vi "MakePhiAxis (SubVI).vi"(2 "radialBinAxis":dbl[](array[numeric]), 3 "angular pixel \ncoverage factor":dbl) -> (15 "lengths":i32[](array[numeric]), 16 "Rsin(phi)[Q]":dbl[][][](array[numeric]), 17 "Rcos(phi)[Q]":dbl[][][](array[numeric]))   [LabVIEW 2011, in "OfflineTracker.lvlib"]
uses:
  OfflineTracker.lvlib
panel:
  out "Waveform Graph":dbl[][](graph)
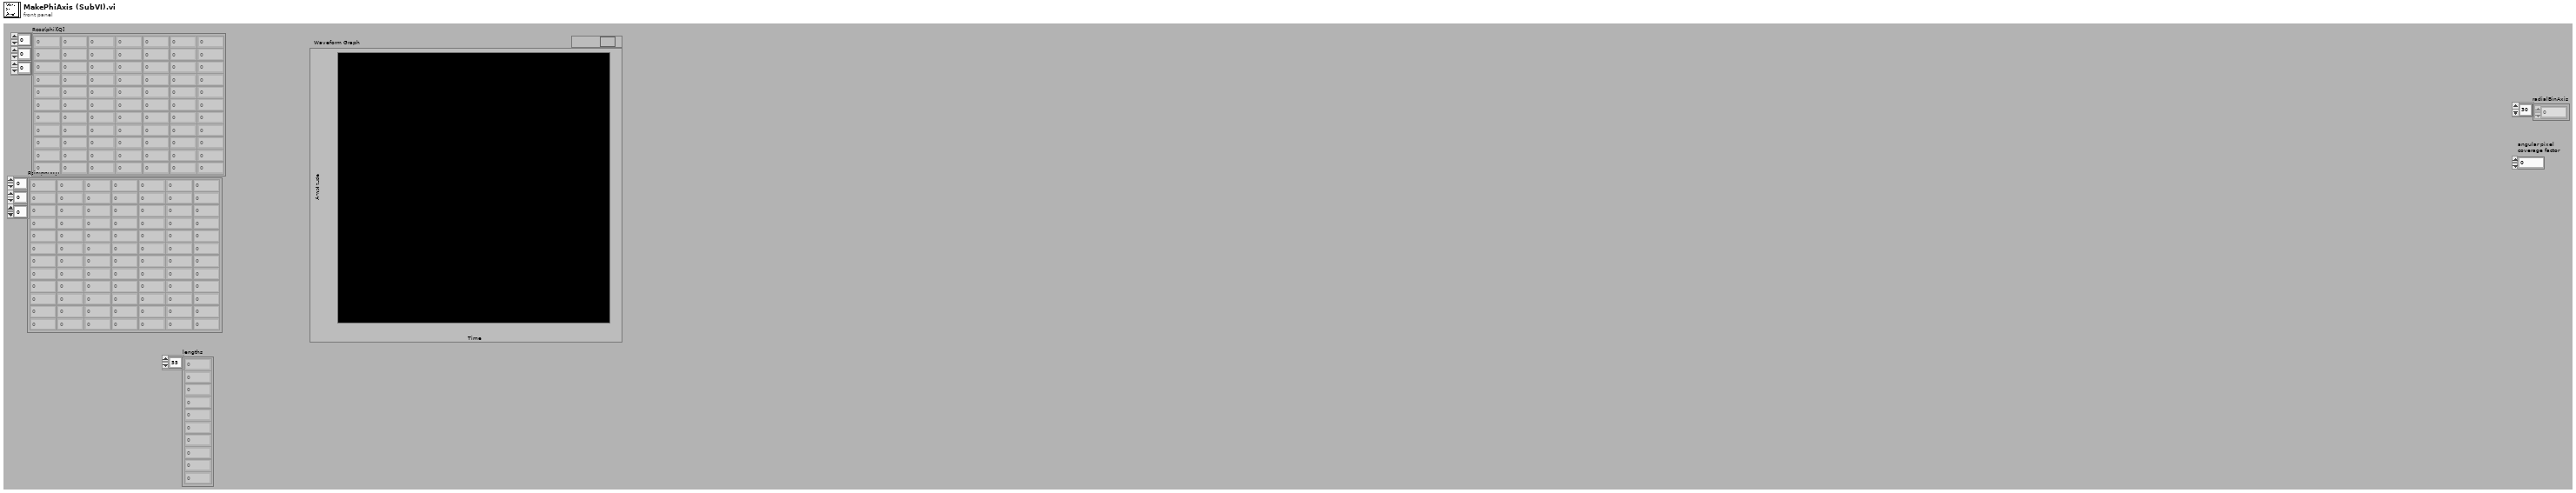
[diagram p1: front panel]
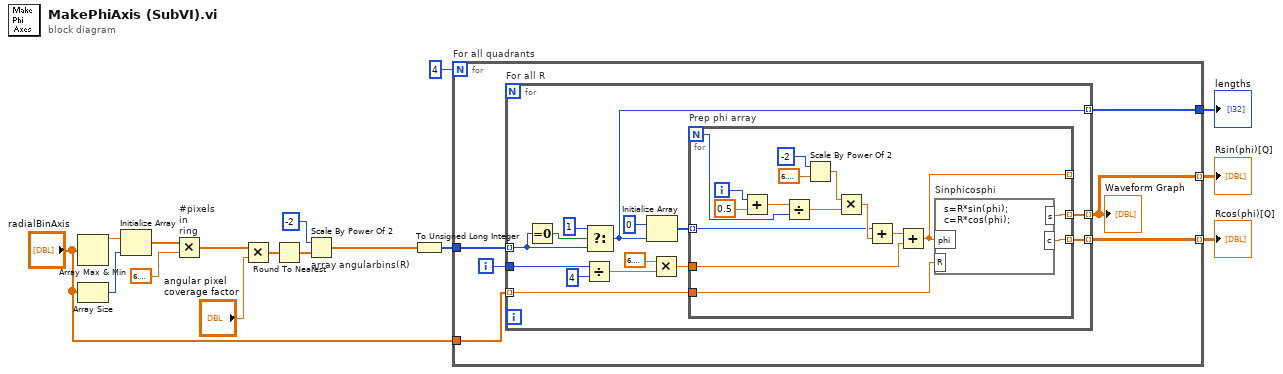
[diagram p0: block diagram]
diagram:
  n1 = Array Max & Min(array="radialBinAxis") -> (max value=w2:dbl)  [unwired: 3 out]
  n2 = Array Size(array="radialBinAxis") -> (size(s)=w3:i32)
  n3 = Initialize Array(w2, w3) -> (w1:dbl[])
  n4 = Multiply "#pixels\nin\nring"(x=w1, y=6.283185307179586) -> (x*y=w9:dbl[])
  n5 = Multiply(x=w9, y="angular pixel \ncoverage factor") -> (x*y=w8:dbl[])
  n6 = Round To Nearest(number=w8) -> (nearest integer value=w7:dbl[])
  n7 = Scale By Power Of 2 "array angularbins(R)"(n=-2, x=w7) -> (x*2^n=w14:dbl[])
  n8 = To Unsigned Long Integer(number=w14) -> (unsigned 32bit integer=w6:u32[])
  n9 = for "For all quadrants" {
    N: 4 -> [_]
    tunnel: w6 -> [w22]
    tunnel: [w19] -> w10 mode=indexing
    tunnel: [w21] -> w11 mode=indexing
    tunnel: "radialBinAxis" -> [w20]
    tunnel: [w17] -> w5
    i -> [w18]
    n10 = for "For all R" {
      tunnel: w22 -> [w24] mode=indexing
      tunnel: [w29] -> w21 mode=indexing
      tunnel: [w30] -> w19 mode=indexing
      tunnel: w18 -> [w28]
      tunnel: w20 -> [w27] mode=indexing
      tunnel: [w23] -> w17 mode=indexing
      n11 = Equal To 0?(x=w24) -> (x = 0?=w26:bool)
      n12 = Divide(x=w28, y=4) -> (x/y=w35:dbl)
      n13 = Select(t=u32 1, s=w26, f=w24) -> (s? t:f=w23:u32)
      n14 = Initialize Array(0 ("element"), w23) -> (w32:i32[])
      n15 = Multiply(x=6.283185307179586, y=w35) -> (x*y=w36:dbl)
      n16 = for "Prep phi array" {
        N -> [w52]
        tunnel: w32 -> [w40] mode=indexing
        tunnel: [w44] -> _ mode=indexing
        tunnel: w36 -> [w47]
        tunnel: [w43] -> w30 mode=indexing
        tunnel: [w42] -> w29 mode=indexing
        tunnel: w27 -> [w37]
        i -> [w39]
        n17 = Add(x=w39, y=0.5) -> (x+y=w38:dbl)
        n18 = Divide(x=w38, y=w52) -> (x/y=w51:dbl)
        n19 = Scale By Power Of 2(n=-2, x=6.283185307179586) -> (x*2^n=w49:dbl)
        n20 = Multiply(x=w49, y=w51) -> (x*y=w50:dbl)
        n21 = Add(x=w40, y=w50) -> (x+y=w48:dbl)
        n22 = Add(x=w48, y=w47) -> (x+y=w44:dbl)
        n23 = formula code="s=R*sin(phi);\nc=R*cos(phi);" "Sinphicosphi"("phi"=w44, "R"=w37) -> ("s"=w43:dbl, "c"=w42:dbl)
      }
    }
    "Waveform Graph" <- w19
  }
  "lengths" <- w5
  "Rsin(phi)[Q]" <- w10
  "Rcos(phi)[Q]" <- w11
